vi "Msg.vi"(7 "Actor in":refnum<class "Actor.lvclass">, 11 "Destroy Msg in":refnum<class "Destroy Msg.lvclass">) -> (5 "Actor out":refnum<class "Actor.lvclass">)   [LabVIEW 2021, in "Destroy.lvlib" / "Destroy Msg.lvclass"]
uses:
  Destroy Msg.lvclass
  Actor/Actor.lvclass
  Destroy/Destroy.lvclass
  8b074ebc-55b2-44bc-a317-0de79f881938.vi
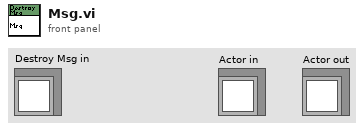
[diagram p1: front panel]
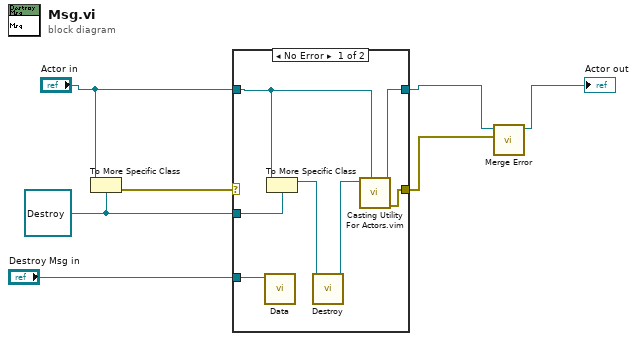
[diagram p0: block diagram]
diagram:
  w4 = refnum<class "Destroy.lvclass"> refnum ("Destroy.lvlib:Destroy.lvclass")
  n1 = To More Specific Class(target class=w4, reference="Actor in") -> (error out=w7:errorcluster)  [unwired: 1 in, 1 out]
  n2 = case shown="No Error" w7 {
    selector: w7 -> [_ w15]
    tunnel: [w13 w16] -> w3
    tunnel: "Actor in" -> [w12 w16]
    tunnel: w4 -> [w14 _]
    tunnel: "Destroy Msg in" -> [w11 _]
    tunnel: [w8 w15] -> w1
    frame No Error {
      n3 = call "Data.vi"("Destroy Msg in"=w11) -> ()  [unwired: 11 in]
      n4 = To More Specific Class(target class=w14, reference=w12) -> (specific class reference=w10:refnum<class "Destroy.lvclass">)  [unwired: 1 in, 1 out]
      n5 = call-dynamic "Destroy.vi"("Destroy in"=w10) -> ("Destroy out"=w9:refnum<class "Destroy.lvclass">)  [unwired: 10 in]
      n6 = call "Casting Utility For Actors.vim"("type"=w12, "Actor in"=w9) -> ("error out"=w8:errorcluster, "Actor out"=w13:refnum<class "Actor.lvclass">)  [unwired: 8 in]
    }
    frame Error {
    }
  }
  n7 = call-dynamic "Merge Error.vi"("Error"=w1, "Set Error in"=w3) -> ("Set Error out"=→"Actor out":refnum<class "Actor.lvclass">)  [unwired: 9 in]
